vi "GetCurrent.vi"(4 "error in":errorcluster, 5 "connection ID":refnum<k5>) -> (0 "Current":string, 1 "error out":errorcluster, 2 "connection ID out":refnum<k5>, 3 "Answer":bool)   [LabVIEW 2013]
panel:
  out "читаю hex":string
  out "читаю текст":string
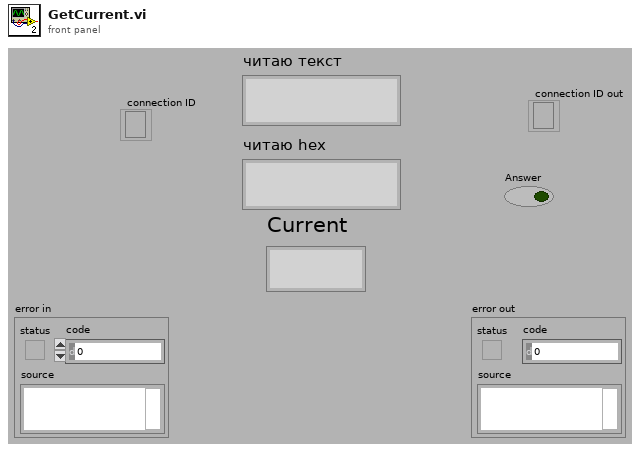
[diagram p1: front panel]
types:
  T1 = enum16{"Standard", "Buffered", "CRLF", "Immediate"}
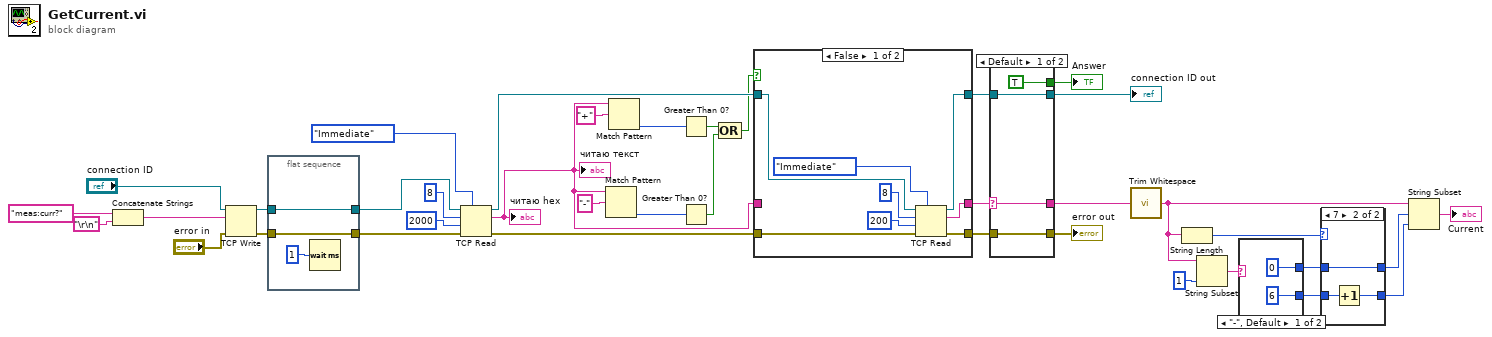
[diagram p0: block diagram]
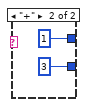
[diagram p3: hidden frame]
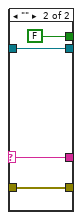
[diagram p5: hidden frame]
diagram:
  n1 = Concatenate Strings("meas:curr?" ("data in"), "\r\n") -> (w35:string)
  n2 = TCP Write(connection ID="connection ID", data in=w35, error in (no error)="error in") -> (connection ID out=w29:refnum<k5>, error out=w31:errorcluster)  [unwired: 2 out]
  n3 = flat-sequence {
    tunnel: [w41] -> w30
    tunnel: w31 -> [w41]
    tunnel: [w40] -> w28
    tunnel: w29 -> [w40]
    frame #0 {
      n4 = Wait (ms)(milliseconds to wait=u32 1) -> ()  [unwired: 1 out]
    }
  }
  n5 = TCP Read(connection ID=w28, bytes to read=8, error in (no error)=w30, 7:T1."Immediate" ("mode (standard)"), 9:2000 ("timeout ms (25000)")) -> (connection ID out=w20:refnum<k5>, data out=w14:string, error out=w18:errorcluster)
  "читаю hex" <- w14
  "читаю текст" <- w14
  n6 = Match Pattern(string=w14, regular expression="-") -> (offset past match=w15:i32)  [unwired: 1 in, 3 out]
  n7 = Match Pattern(string=w14, regular expression="+") -> (offset past match=w26:i32)  [unwired: 1 in, 3 out]
  n8 = Greater Than 0?(x=w26) -> (x > 0?=w13:bool)
  n9 = Greater Than 0?(x=w15) -> (x > 0?=w12:bool)
  n10 = Compound Arithmetic op=OR(w13, w12) -> (w11:bool)
  n11 = case shown="False" w11 {
    tunnel: w14 -> [_ w52]
    tunnel: [w42 w52] -> w21
    tunnel: w20 -> [w46 w51]
    tunnel: [w45 w51] -> w19
    tunnel: w18 -> [w44 w50]
    tunnel: [w43 w50] -> w17
    frame False {
      n12 = TCP Read(connection ID=w46, bytes to read=8, error in (no error)=w44, 7:T1."Immediate" ("mode (standard)"), 9:200 ("timeout ms (25000)")) -> (connection ID out=w45:refnum<k5>, data out=w42:string, error out=w43:errorcluster)
    }
    frame True {
    }
  }
  n13 = case shown="Default" w21 {
    selector: w21 -> [w56 w60]
    tunnel: [w56 w60] -> w9
    tunnel: [TRUE FALSE] -> w22
    tunnel: w17 -> [w54 w58]
    tunnel: [w54 w58] -> w24
    tunnel: w19 -> [w53 w57]
    tunnel: [w53 w57] -> w25
    frame Default {
    }
    frame "" {
    }
  }
  "Answer" <- w22
  "connection ID out" <- w25
  "error out" <- w24
  n14 = call <vilib>:"Trim Whitespace.vi"("string"=w9) -> ("trimmed string"=w6:string)  [unwired: 1 in]
  n15 = String Length(string=w6) -> (length=w5:i32)
  n16 = String Subset(string=w6, length (rest)=1 ("length (rest)")) -> (substring=w8:string)  [unwired: 1 in]
  n17 = case shown="\"-\", Default" w8 {
    tunnel: [0 ("length (rest)") 1 ("length (rest)")] -> w2
    tunnel: [6 ("length (rest)") 3 ("length (rest)")] -> w4
    frame "-", Default {
    }
    frame "+" {
    }
  }
  n18 = case shown="7" w5 {
    tunnel: w4 -> [w66 w69]
    tunnel: [w66 w68] -> w3
    tunnel: w2 -> [w65 w67]
    tunnel: [w65 w67] -> w1
    frame 6, Default {
    }
    frame 7 {
      n19 = Increment(x=w69) -> (x+1=w68:i32)
    }
  }
  n20 = String Subset(string=w6, offset (0)=w1, length (rest)=w3) -> (substring=→"Current":string)
